vi "filtro.vi"(11 "Boolean out 1":bool) -> (3 "Boolean":bool)   [LabVIEW 2017]
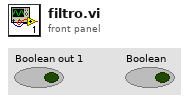
[diagram p1: front panel]
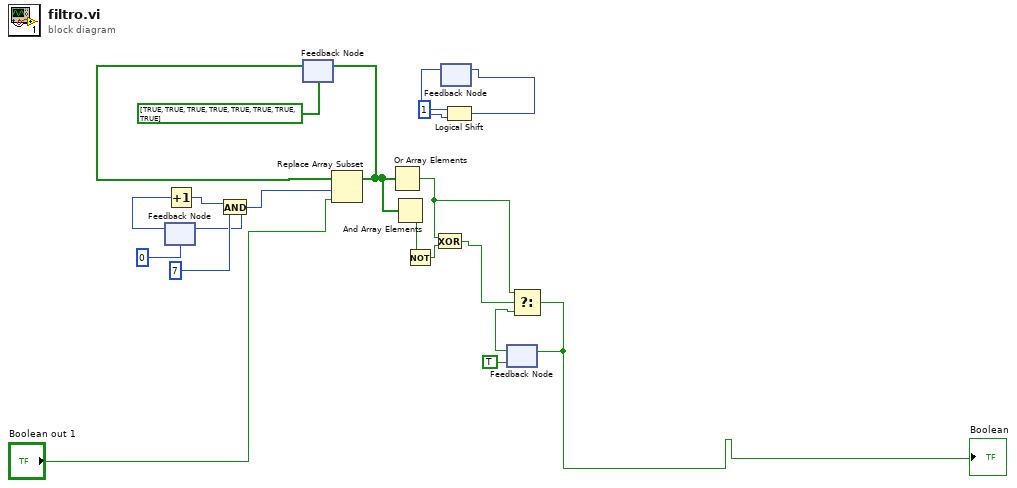
[diagram p0: block diagram]
diagram:
  n1 = feedback #1(u8 0) -> (w4:u8)
  n2 = Increment(x=w4) -> (x+1=w3:u8)
  n3 = And(x=w3, y=u8 7) -> (x .and. y?=w2:u8)
  n4 = feedback-in #1(w2) -> ()
  n5 = feedback #2(bool[] [TRUE, TRUE, TRUE, TRUE, TRUE, TRUE, TRUE, TRUE]) -> (w1:bool[])
  n6 = Replace Array Subset(array=w1, new element="Boolean out 1", index=w2) -> (w13:bool[])
  n7 = feedback-in #2(w13) -> ()
  n8 = Or Array Elements(Boolean array=w13) -> (logical OR=w15:bool)
  n9 = And Array Elements(Boolean array=w13) -> (logical AND=w10:bool)
  n10 = Not(x=w10) -> (.not. x?=w11:bool)
  n11 = Exclusive Or(1:w11, 2:w15) -> (0:w14:bool)
  n12 = feedback #3() -> (w7:i16)  [unwired: 1 in]
  n13 = Logical Shift(y=i16 1, x=w7) -> (x << y=w8:i16)
  n14 = feedback-in #3(w8) -> ()
  n15 = feedback #4(TRUE) -> (w18:bool)
  n16 = Select(t=w15, s=w14, f=w18) -> (s? t:f=w17:bool)
  "Boolean" <- w17
  n17 = feedback-in #4(w17) -> ()
